vi "ingresaMediciones.vi"(6 "New Value":string[][](array[string]), 7 "Tbl Refnum":refnum<vi>, 8 "error in (no error)":errorcluster, 9 "mediciones in":T1, 10 "Tabla in":string[][](array[string])) -> (0 "error out":errorcluster, 1 "mediciones out":T1, 2 "Tabla out":string[][](array[string]), 3 "Prueba04 out":refnum<class "Prueba04.lvclass">)   [LabVIEW 2019, in "Prueba04.lvclass"]
uses:
  Prueba04.lvclass
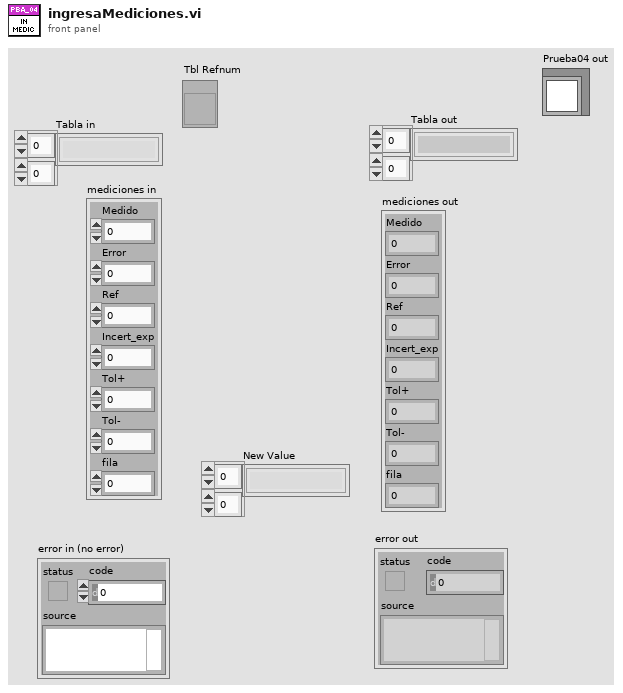
[diagram p1: front panel]
types:
  T1 = cluster{"Medido":dbl, "Error":dbl, "Ref":dbl, "Incert_exp":dbl, "Tol+":dbl, "Tol-":dbl, "fila":i32}
  T2 = typedef "LVRowAndColumnTypeDef.ctl" = cluster{"Row":i32, "Column":i32}
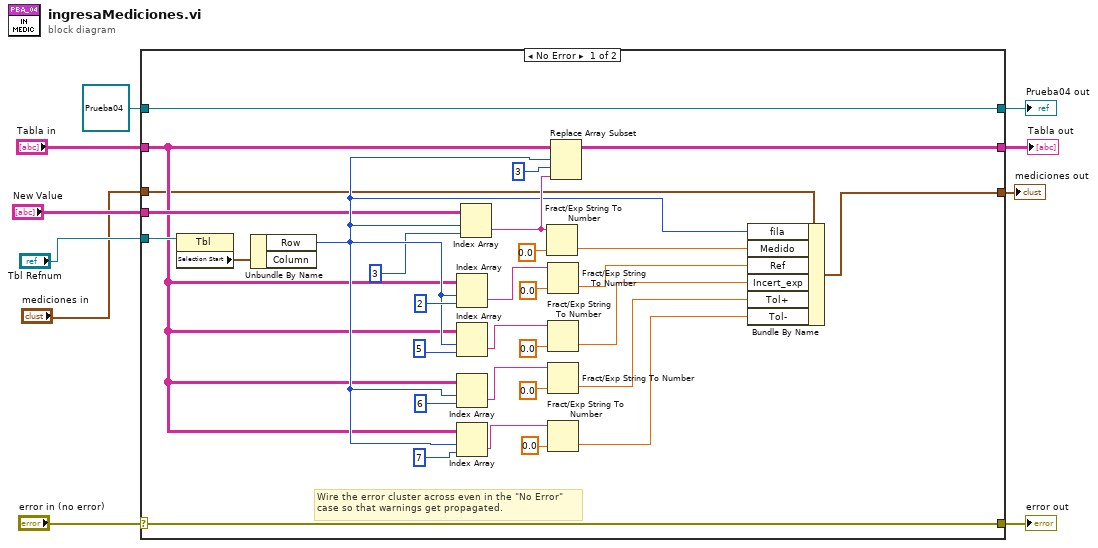
[diagram p0: block diagram]
diagram:
  n1 = case shown="No Error" "error in (no error)" {
    selector: "error in (no error)" -> [w40 w45]
    tunnel: [w40 w45] -> w9
    tunnel: [w41 w44] -> w7
    tunnel: refnum<class "Prueba04.lvclass"> refnum ("Prueba04 in") -> [w41 w44]
    tunnel: "Tabla in" -> [w15 w43]
    tunnel: "New Value" -> [w18 _]
    tunnel: "Tbl Refnum" -> [w17 _]
    tunnel: "mediciones in" -> [w14 w42]
    tunnel: [w13 w43] -> w3
    tunnel: [w12 w42] -> w1
    frame No Error {
      # "Wire the error cluster across even in the \"No Error\"\ncase so that warnings get propagated."
      n2 = property on="Property Node" class="Tbl"(reference=w17) -> ("Selection Start"=w16:T2)  [unwired: 1 in, 2 out]
      n3 = Unbundle By Name(w16) -> ("Row"=w19:i32)  [unwired: 1 out]
      n4 = Index Array(array=w15, index (row)=w19, index (col)=2 ("disabled index (col)")) -> (element=w35:string)
      n5 = Index Array(array=w15, index (row)=w19, index (col)=5 ("index (row)")) -> (element=w30:string)
      n6 = Index Array(array=w15, index (row)=w19, index (col)=6 ("disabled index (col)")) -> (element=w21:string)
      n7 = Index Array(array=w15, index (row)=w19, index (col)=7 ("index (row)")) -> (element=w24:string)
      n8 = Index Array(array=w18, index (row)=w19, index (col)=3) -> (element=w20:string)
      n9 = Fract/Exp String To Number(string=w20, default (0 dbl)=0.0) -> (number=w36:dbl)  [unwired: 2 in, 1 out]
      n10 = Fract/Exp String To Number(string=w35, default (0 dbl)=0.0) -> (number=w34:dbl)  [unwired: 2 in, 1 out]
      n11 = Fract/Exp String To Number(string=w30, default (0 dbl)=0.0) -> (number=w29:dbl)  [unwired: 2 in, 1 out]
      n12 = Fract/Exp String To Number(string=w21, default (0 dbl)=0.0) -> (number=w22:dbl)  [unwired: 2 in, 1 out]
      n13 = Fract/Exp String To Number(string=w24, default (0 dbl)=0.0) -> (number=w23:dbl)  [unwired: 2 in, 1 out]
      n14 = Replace Array Subset(array=w15, new element=w20, index (row)=w19, index (col)=3 ("disabled index (col)")) -> (w13:string[][])
      n15 = Bundle By Name(cluster=w14, "fila"=w19, "Medido"=w36, "Ref"=w34, "Incert_exp"=w29, "Tol+"=w22, "Tol-"=w23) -> (w12:T1)
    }
    frame Error {
    }
  }
  "error out" <- w9
  "Prueba04 out" <- w7
  "Tabla out" <- w3
  "mediciones out" <- w1
